vi "Bairstow_Calculate ds&dr.vi"(10 "C":dbl[](array[numeric]), 11 "B":dbl[](array[numeric])) -> (2 "dr":dbl, 3 "ds":dbl)   [LabVIEW 2010, in "NI_AALPro.lvlib"]
uses:
  NI_AALPro.lvlib
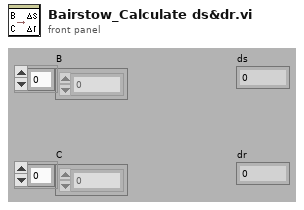
[diagram p1: front panel]
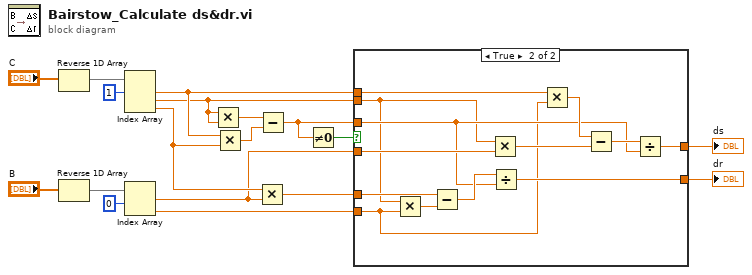
[diagram p0: block diagram]
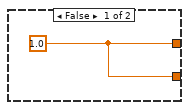
[diagram p2: hidden frame]
diagram:
  n1 = Reverse 1D Array(array="C") -> (reversed array=w14:dbl[])
  n2 = Reverse 1D Array(array="B") -> (reversed array=w16:dbl[])
  n3 = Index Array(array=w14, index #1=1 ("index")) -> (element #1=w8:dbl, element #2=w6:dbl, element #3=w10:dbl)  [unwired: 2 in]
  n4 = Index Array(array=w16, index #1=0 ("index")) -> (element #1=w5:dbl, element #2=w7:dbl)  [unwired: 1 in]
  n5 = Multiply(x=w6, y=w6) -> (x*y=w12:dbl)
  n6 = Multiply(x=w8, y=w10) -> (x*y=w11:dbl)
  n7 = Multiply(x=w10, y=w5) -> (x*y=w9:dbl)
  n8 = Subtract(x=w12, y=w11) -> (x-y=w1:dbl)
  n9 = Not Equal To 0?(x=w1) -> (x != 0?=w2:bool)
  n10 = case shown="True" w2 {
    tunnel: w9 -> [_ w32]
    tunnel: w8 -> [_ w30]
    tunnel: w7 -> [_ w21]
    tunnel: w6 -> [_ w20]
    tunnel: w5 -> [_ w29]
    tunnel: [w19 w26] -> w4
    tunnel: w1 -> [_ w23]
    tunnel: [w19 w22] -> w3
    frame False {
      w19 = 1.0
    }
    frame True {
      n11 = Multiply(x=w20, y=w21) -> (x*y=w31:dbl)
      n12 = Subtract(x=w32, y=w31) -> (x-y=w25:dbl)
      n13 = Multiply(x=w20, y=w29) -> (x*y=w27:dbl)
      n14 = Divide(x=w25, y=w23) -> (x/y=w22:dbl)
      n15 = Multiply(x=w30, y=w21) -> (x*y=w28:dbl)
      n16 = Subtract(x=w28, y=w27) -> (x-y=w24:dbl)
      n17 = Divide(x=w24, y=w23) -> (x/y=w26:dbl)
    }
  }
  "ds" <- w4
  "dr" <- w3
